vi "Download to Cache.vi"(7 "Force Refresh? (F)":bool, 8 "error in (no error)":errorcluster, 11 "URL":string) -> (0 "error out":errorcluster, 1 "last mod":timestamp, 2 "From Cache?":bool, 3 "Cache Path":path)   [LabVIEW 2020, in "GCentral-API.lvlib"]
uses:
  GCentral-API.lvlib
  neg-pkg/URI/URI.lvclass
  <vilib>/httpClient/LabVIEWHTTPClient.lvlib
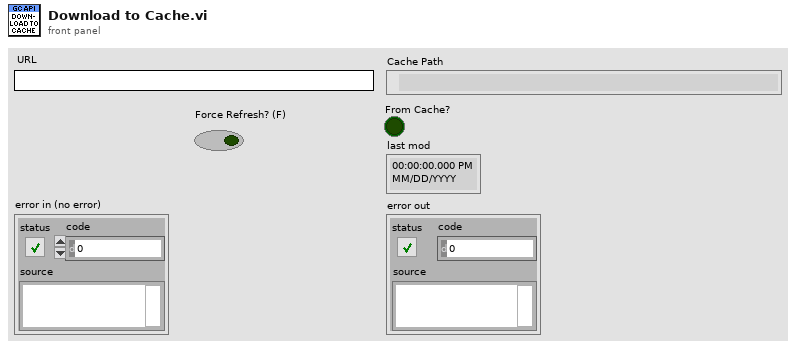
[diagram p1: front panel]
types:
  T1 = typedef "LabVIEWHTTPClient.lvlib/ClientHandle.ctl" = refnum<k1>
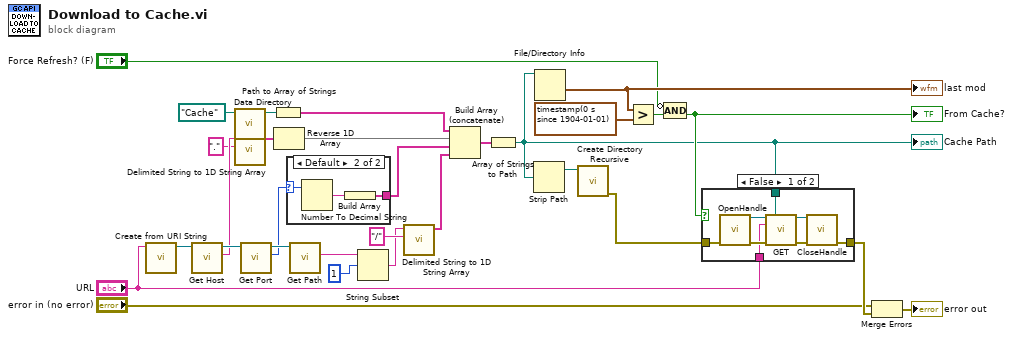
[diagram p0: block diagram]
diagram:
  n1 = call "Create from URI String.vi"("URI String"="URL") -> ("URI out"=w30:refnum<class "URI.lvclass">)  [unwired: 9 in, 1 out]
  n2 = call "Get Host.vi"("URI in"=w30) -> ("Host"=w27:string, "URI out"=w29:refnum<class "URI.lvclass">)  [unwired: 8 in, 1 out]
  n3 = call "Data Directory.vi"("Subfolder (None)"=path "Cache") -> ("GCentral Data"=w20:path)  [unwired: 10 in]
  n4 = call <vilib>:"Delimited String to 1D String Array.vi"("delimiter"=".", "delimited string"=w27) -> ("string array"=w25:string[])  [unwired: 9 in]
  n5 = call "Get Port.vi"("URI in"=w29) -> ("Port"=w22:u16, "URI out"=w28:refnum<class "URI.lvclass">)  [unwired: 8 in, 1 out]
  n6 = Path to Array of Strings(0:w20) -> (2:w19:string[])  [unwired: 1 out]
  n7 = Reverse 1D Array(array=w25) -> (reversed array=w23:string[])
  n8 = case shown="Default" w22 {
    selector: w22 -> [_ w33]
    tunnel: [_ w31] -> w15
    frame 0 {
    }
    frame Default {
      n9 = Number To Decimal String(number=w33) -> (decimal integer string=w32:string)  [unwired: 1 in]
      n10 = Build Array(w32) -> (w31:string[])
    }
  }
  n11 = call "Get Path.vi"("URI in"=w28) -> ("Path"=w18:string)  [unwired: 8 in, 2 out]
  n12 = String Subset(string=w18, offset (0)=1) -> (substring=w16:string)  [unwired: 1 in]
  n13 = call <vilib>:"Delimited String to 1D String Array.vi"("delimiter"="/", "delimited string"=w16) -> ("string array"=w13:string[])  [unwired: 9 in]
  n14 = Build Array (concatenate)(w19, w23, w15, w13) -> (w14:string[])
  n15 = Array of Strings to Path(0:w14) -> (2:w3:path)  [unwired: 1 in]
  "Cache Path" <- w3
  n16 = Strip Path(path=w3) -> (stripped path=w2:path)  [unwired: 1 out]
  n17 = File/Directory Info(path=w3) -> (last mod=w12:timestamp)  [unwired: 1 in, 6 out]
  "last mod" <- w12
  n18 = call <vilib>:"Create Directory Recursive.vi"("directory"=w2) -> ("error out"=w1:errorcluster)  [unwired: 4 in, 2 out]
  n19 = Greater?(x=w12, y=timestamp(0 s since 1904-01-01)) -> (0:w9:bool)
  n20 = Compound Arithmetic op=AND(invert "Force Refresh? (F)", w9) -> (w5:bool)
  "From Cache?" <- w5
  n21 = case shown="False" w5 {
    tunnel: "URL" -> [w37 _]
    tunnel: w3 -> [w36 _]
    tunnel: [w35 _] -> w8
    tunnel: w1 -> [w34 _]
    frame False {
      n22 = call <vilib>:"OpenHandle.vi"("error in (no error)"=w34) -> ("client handle out"=w41:T1, "error out"=w40:errorcluster)  [unwired: 13 in]
      n23 = call <vilib>:"GET.vi"("client handle"=w41, "output file"=w36, "url"=w37, "error in (no error)"=w40) -> ("client handle out"=w38:T1, "error out"=w39:errorcluster)  [unwired: 8 in, 2 out]
      n24 = call <vilib>:"CloseHandle.vi"("client handle"=w38, "error in (no error)"=w39) -> ("error out"=w35:errorcluster)  [unwired: 13 in]
    }
    frame True {
    }
  }
  n25 = Merge Errors("error in (no error)", w8) -> (→"error out":errorcluster)
